vi "List Channels by Classification.vi"(11 "E2E configuration in":refnum<class "E2E Tag Exchange configuration.lvclass">) -> (1 "Output Channels":refnum<class "TBM channel.lvclass">[](array[class]), 2 "Input Channels":refnum<class "TBM channel.lvclass">[](array[class]), 3 "E2E configuration out":refnum<class "E2E Tag Exchange configuration.lvclass">)   [LabVIEW 2015, in "E2E Tag Exchange configuration.lvclass"]
uses:
  E2E Tag Exchange configuration.lvclass
  <vilib>/NI/Tag Bus Module Framework/channel/TBM channel.lvclass
  <vilib>/NI/Tag Bus Module Framework/channel/channel classification.ctl
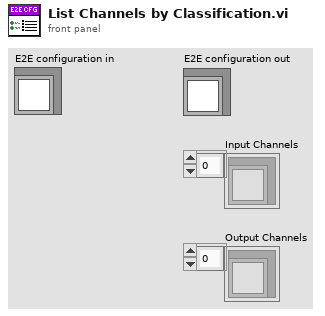
[diagram p1: front panel]
types:
  T1 = typedef "TBM channel.lvclass/channel classification.ctl" = enum16{"input data", "output data", "processing parameter", "processing result"}
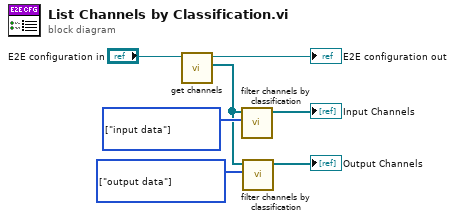
[diagram p0: block diagram]
diagram:
  w5 = T1[] [enum."output data"] items=["input data", "output data", "processing parameter", "processing result"] ("allowed classifications")
  w4 = T1[] [enum."input data"] items=["input data", "output data", "processing parameter", "processing result"] ("allowed classifications")
  n1 = call-dynamic "get channels.vi"("E2E configuration in"="E2E configuration in") -> ("channels"=w3:refnum<class "TBM channel.lvclass">[], "E2E configuration out"=→"E2E configuration out":refnum<class "E2E Tag Exchange configuration.lvclass">)  [unwired: 9 in]
  n2 = call <vilib>:"filter channels by classification.vi"("allowed classifications"=w4, "channels in"=w3) -> ("channels out"=→"Input Channels":refnum<class "TBM channel.lvclass">[])  [unwired: 9 in]
  n3 = call <vilib>:"filter channels by classification.vi"("allowed classifications"=w5, "channels in"=w3) -> ("channels out"=→"Output Channels":refnum<class "TBM channel.lvclass">[])  [unwired: 9 in]
